vi "年月日字符串转时间单位.vi"(11 "年月日字符串":string) -> (3 "time stamp":timestamp)   [LabVIEW 2014]
uses:
  <vilib>/Utility/miscctls.llb/LVDateTimeRec.ctl
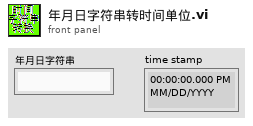
[diagram p1: front panel]
types:
  T1 = typedef "LVDateTimeRec.ctl" = cluster{"fractional second":dbl, "second":i32, "minute":i32, "hour":i32, "day of month":i32, "month":i32, "year":i32, "day of week":i32, "day of year":i32, "DST":i32}
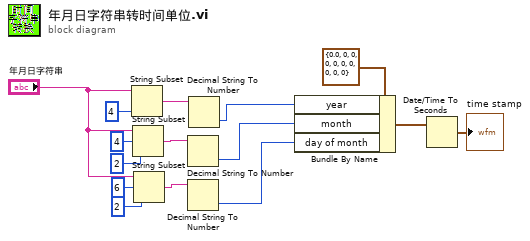
[diagram p0: block diagram]
diagram:
  n1 = String Subset(string="年月日字符串", length (rest)=4 ("长度（剩余）")) -> (substring=w10:string)  [unwired: 1 in]
  n2 = String Subset(string="年月日字符串", offset (0)=4 ("偏移量(0)"), length (rest)=2 ("长度（剩余）")) -> (substring=w11:string)
  n3 = String Subset(string="年月日字符串", offset (0)=6 ("偏移量(0)"), length (rest)=2 ("长度（剩余）")) -> (substring=w12:string)
  n4 = Decimal String To Number(string=w11) -> (number=w14:i32)  [unwired: 2 in, 1 out]
  n5 = Decimal String To Number(string=w12) -> (number=w15:i32)  [unwired: 2 in, 1 out]
  n6 = Decimal String To Number(string=w10) -> (number=w13:i32)  [unwired: 2 in, 1 out]
  n7 = Bundle By Name(cluster=T1 {"fractional second"=0.0, "second"=0, "minute"=0, "hour"=0, "day of month"=0, "month"=0, "year"=0, "day of week"=0, "day of year"=0, "DST"=0} ("日期时间记录 2"), "year"=w13, "month"=w14, "day of month"=w15) -> (w7:T1)
  n8 = Date/Time To Seconds(2:w7) -> (0:→"time stamp":timestamp)  [unwired: 1 in]
